vi "2L11_Init_N.vi"(1 "ni":u32[](array[numeric])) -> ()   [LabVIEW 2010, in "lv_02.lvlib"]
uses:
  lv_02.lvlib
panel:
  out "OBS/MIF":enum16{"OBS", "MIF"}(ring)
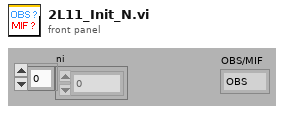
[diagram p1: front panel]
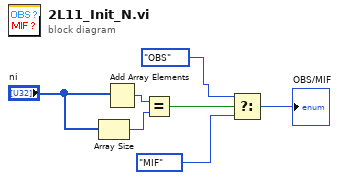
[diagram p0: block diagram]
diagram:
  n1 = Array Size(array="ni") -> (size(s)=w5:i32)
  n2 = Add Array Elements(numeric array="ni") -> (sum=w4:u32)
  n3 = Equal?(x=w4, y=w5) -> (x = y?=w7:bool)
  n4 = Select(t=enum16{"OBS", "MIF"}."OBS" ("OBS/MIF"), s=w7, f=enum16{"OBS", "MIF"}."MIF" ("OBS/MIF")) -> (s? t:f=→"OBS/MIF":enum16{"OBS", "MIF"})
